vi "gyro app -- V1.vi"() -> ()   [LabVIEW 2020]
uses:
  launch items list.ctl
  pll internal user event action.ctl
  que event bag action.ctl
  server talkto message type.ctl
  server talkback message type.ctl
  cursor action.ctl
panel:
  in  "Main":enum32{"all"}(tab)
  in  "exit!":bool=TRUE
  in  "processes":cluster{"item":T1, "gear":bool}[](array[cluster])=[{"item"=enum."source", "gear"=FALSE}, {"item"=enum."fitter", "gear"=FALSE}, {"item"=enum."sweeper engine", "gear"=FALSE}, {"item"=enum."sweeper monitor", "gear"=FALSE}, {"item"=enum."pll engine", "gear"=FALSE}, {"item"=enum."pll monitor", "gear"=FALSE}]
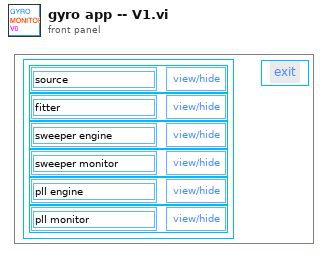
[diagram p1: front panel]
types:
  T1 = typedef "launch items list.ctl" = enum16{"source", "pll engine", "pll monitor", "sweeper engine", "sweeper monitor", "fitter"}
  T2 = typedef "pll internal user event action.ctl" = enum16{"gear pll engine", "start pll async", "stop pll async", "toggle pll async", "gear sweeper", "start sweeper", "stop sweeper", "toggle sweeper", "accept frequency", "reset lorentzian", "accept lorentzian", "update cursors", "pause pll", "unpause pll", "void", "exit", "gear sweeper monitor", "gear sweeper engine", "gear fitter", "gear sourcer", "gear pll monitor"}
  T3 = typedef "que event bag action.ctl" = enum16{"check", "add", "init", "keys", "values"}
  T4 = typedef "server talkback message type.ctl" = cluster{"message":enum16{"new", "void"}}
  T5 = typedef "server talkto message type.ctl" = cluster{"message":enum16{"stop", "start", "update pars", "update request", "new", "launch", "exit", "get", "reset", "pause", "unpause"}}
  T6 = typedef "server talk-to-back pair.ctl" = cluster{"talkback event":refnum<user-event>, "talkto event":refnum<user-event>}
  T7 = typedef "cursor action.ctl" = enum16{"range", "read", "write", "check", "zoom out", "smart zoom out", "zoom to aspect ratio 1", "zoom to win", "zoom out 20%", "zoom in 20%", "-empty", "smart zoom out&aspect", "move range left 20%", "move range right 20%", "move range up 20%", "move range down 20%", "zoom to X win", "zoom to Y win", "zoom out X", "zoom out Y", "zoom in X", "zoom in Y", "check plot scale", "set plot color", "set Xlabel", "set Ylabel", "set cursor color"}
  T8 = enum32{"Invalid", "Standard", "Closed", "Hidden", "Minimized", "Maximized"}
  T9 = typedef "eventvkey.ctl" = enum16{"ASCII", "Enter", "Return", "Shift", "Ctrl", "Alt", "Cmd", "Opt", "Caps", "NumLock", "Clear", "Break", "Up", "Down", "Left", "Right", "Insert", "Delete", "Home", "End", "PageUp", "PageDown", "Escape", "Help", "Pause", "ScrollLock", "F1", "F2", "F3", "F4", "F5", "F6", "F7", "F8", "F9", "F10", "F11", "F12", "F13", "F14", "F15", "F16", "F17", "F18", "F19", "F20", "F21", "F22", "F23", "F24", "Play", "VolumeUp", "VolumeDown", "Mute", "Two Byte Char"}
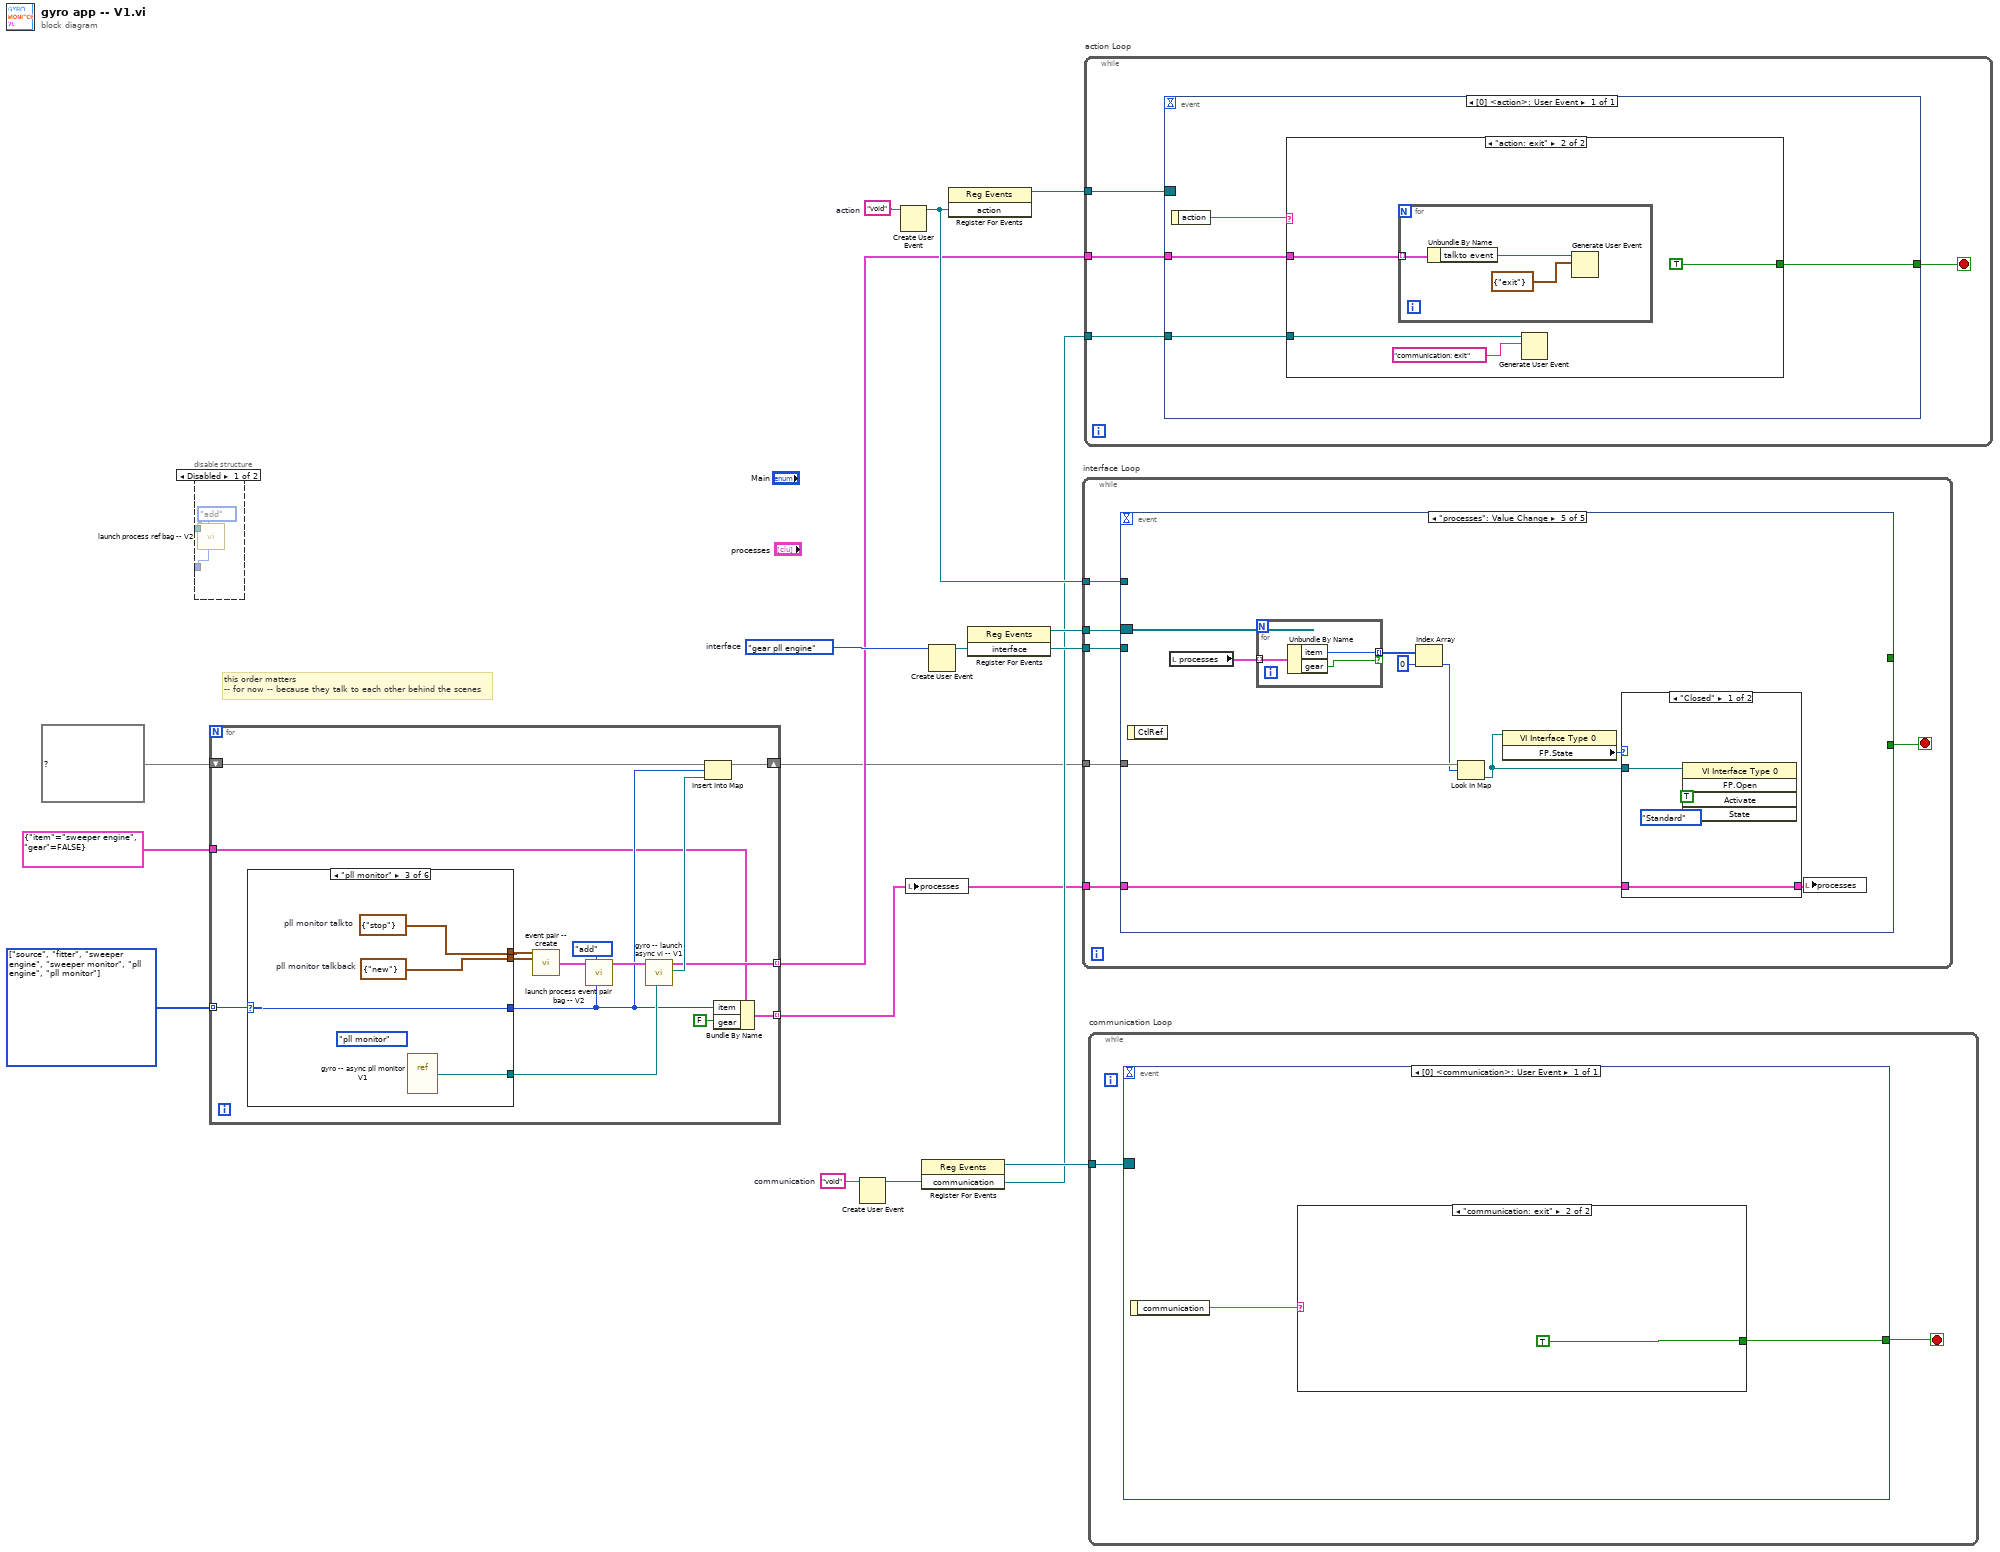
[diagram p0: block diagram]
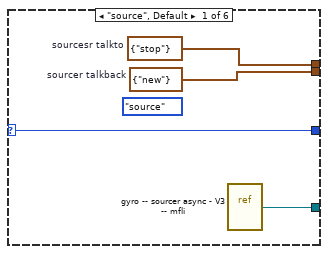
[diagram p3: hidden frame]
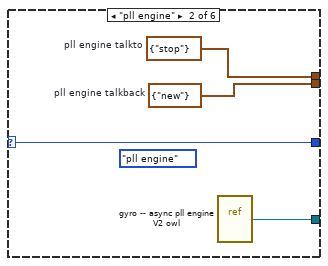
[diagram p4: hidden frame]
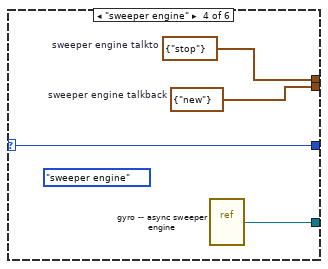
[diagram p5: hidden frame]
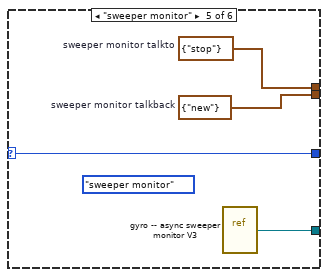
[diagram p6: hidden frame]
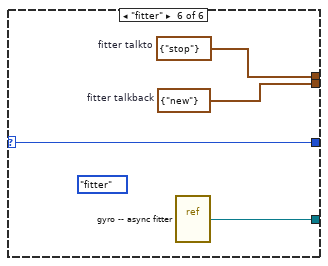
[diagram p7: hidden frame]
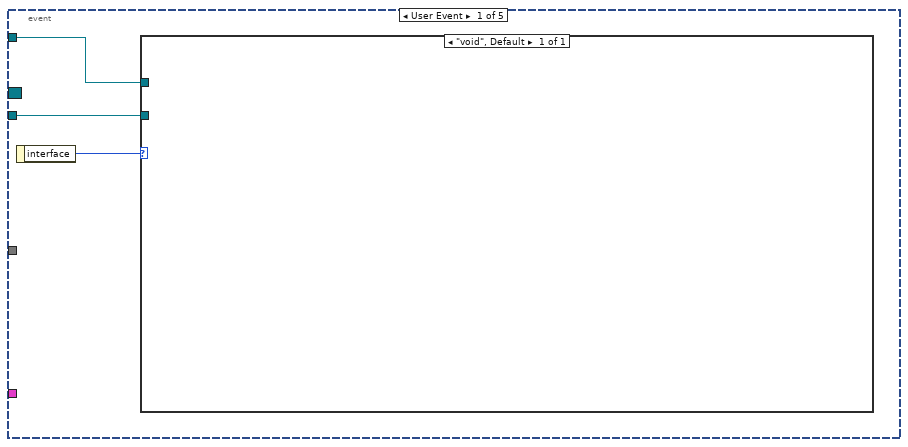
[diagram p10: hidden frame]
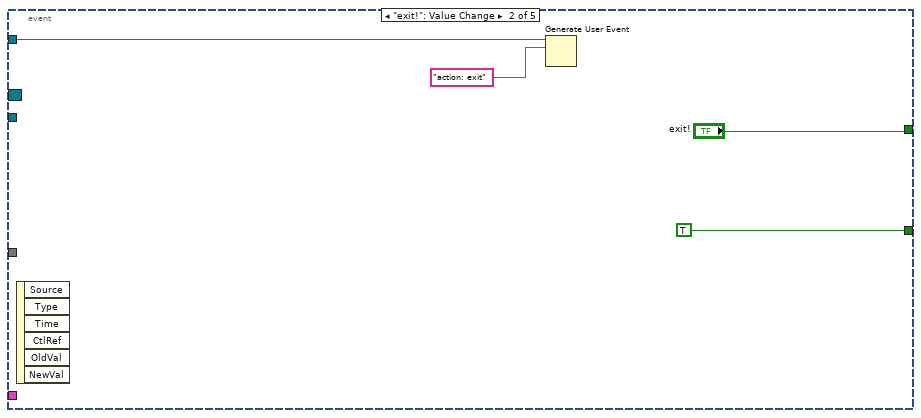
[diagram p11: hidden frame]
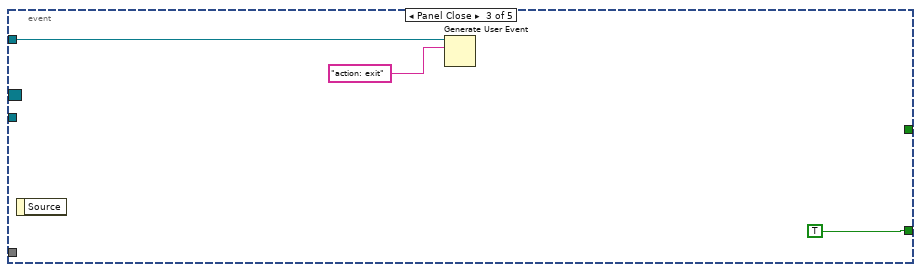
[diagram p12: hidden frame]
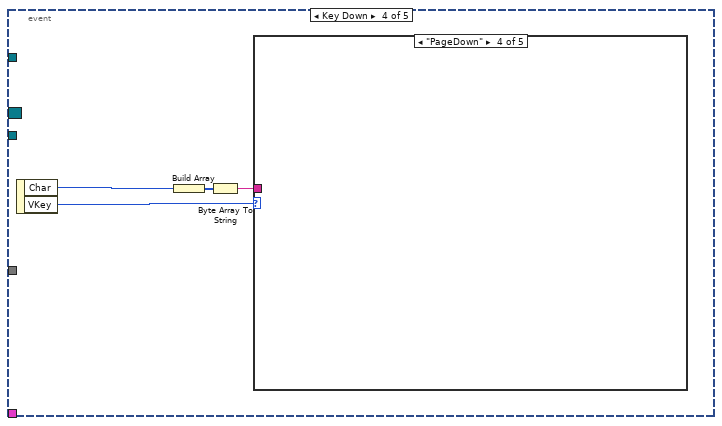
[diagram p13: hidden frame]
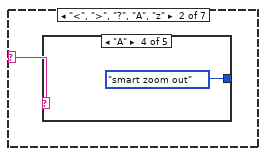
[diagram p16: hidden frame]
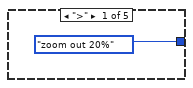
[diagram p17: hidden frame]
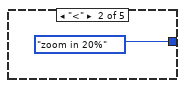
[diagram p18: hidden frame]
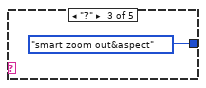
[diagram p19: hidden frame]
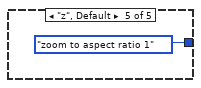
[diagram p20: hidden frame]
diagram:
  w5 = T1[] [enum."source", enum."fitter", enum."sweeper engine", enum."sweeper monitor", enum."pll engine", enum."pll monitor"] items=["source", "pll engine", "pll monitor", "sweeper engine", "sweeper monitor", "fitter"]
  w8 = "void"  # communication
  w11 = "void"  # action
  w13 = pll_internal_user_event_action."gear pll engine"  # interface
  # "this order matters\n-- for now -- because they talk to each other behind the scenes"
  n1 = disable-structure shown="Disabled" {
    disable-tunnel: _ -> [w17 _]
    disable-tunnel: _ -> [w16 _]
    frame Disabled {
      n2 = call "launch process ref bag -- V2.vi"("launch item"=w17, "bag action"=que_event_bag_action."add", "process ref IN"=w16) -> ()  [unwired: 6 in, 3 out]
    }
    frame Enabled {
    }
  }
  n3 = for {
    tunnel: w5 -> [w24] mode=indexing
    tunnel: [w21] -> w7 mode=indexing
    tunnel: [w27] -> w4 mode=indexing
    shift-right: [w25] -> w2
    shift-left: map{T1, refnum<vi>} {} ("Map 2") -> [w26]
    tunnel: cluster{"item":T1, "gear":bool} {"item"=enum."sweeper engine", "gear"=FALSE} ("Cluster") -> [w19]
    n4 = case shown="\"pll monitor\"" w24 {
      selector: w24 -> [w37 w41 w45 w46 w51 w57]
      tunnel: [w35 w39 w43 w49 w53 w56] -> w31
      tunnel: [w34 w38 w42 w48 w52 w55] -> w30
      tunnel: [w37 w41 w45 w46 w51 w57] -> w20
      tunnel: [w36 w40 w44 w47 w50 w54] -> w28
      frame "source", Default {
        (unwired) launch_items_list."source" ("launch items")
        w34 = T4 {"message"=enum."new"}  # sourcer talkback
        w35 = T5 {"message"=enum."stop"}  # sourcesr talkto
        n5 = vi-ref "gyro -- sourcer async - V3 -- mfli.vi"() -> (w36:refnum<vi>)
      }
      frame "pll engine" {
        (unwired) launch_items_list."pll engine" ("launch items")
        w38 = T4 {"message"=enum."new"}  # pll engine talkback
        w39 = T5 {"message"=enum."stop"}  # pll engine talkto
        n6 = vi-ref "gyro -- async pll engine V2 owl.vi"() -> (w40:refnum<vi>)
      }
      frame "pll monitor" {
        (unwired) launch_items_list."pll monitor" ("launch items")
        w42 = T4 {"message"=enum."new"}  # pll monitor talkback
        w43 = T5 {"message"=enum."stop"}  # pll monitor talkto
        n7 = vi-ref "gyro -- async pll monitor V1.vi"() -> (w44:refnum<vi>)
      }
      frame "sweeper engine" {
        (unwired) launch_items_list."sweeper engine" ("launch items")
        w48 = T4 {"message"=enum."new"}  # sweeper engine talkback
        w49 = T5 {"message"=enum."stop"}  # sweeper engine talkto
        n8 = vi-ref "gyro -- async sweeper engine.vi"() -> (w47:refnum<vi>)
      }
      frame "sweeper monitor" {
        (unwired) launch_items_list."sweeper monitor" ("launch items")
        w52 = T4 {"message"=enum."new"}  # sweeper monitor talkback
        w53 = T5 {"message"=enum."stop"}  # sweeper monitor talkto
        n9 = vi-ref "gyro -- async sweeper monitor V3.vi"() -> (w50:refnum<vi>)
      }
      frame "fitter" {
        (unwired) launch_items_list."fitter" ("launch items")
        w55 = T4 {"message"=enum."new"}  # fitter talkback
        w56 = T5 {"message"=enum."stop"}  # fitter talkto
        n10 = vi-ref "gyro -- async fitter.vi"() -> (w54:refnum<vi>)
      }
    }
    n11 = call "event pair -- create.vi"("talkto"=w31, "talkback"=w30) -> ("even pair out"=w29:T6)  [unwired: 11 in, 2 out]
    n12 = call "launch process event pair bag -- V2.vi"("launch item"=w20, "bag action"=que_event_bag_action."add", "event pair IN"=w29) -> ("event pair OUT"=w33:T6)  [unwired: 6 in, 2 out]
    n13 = call "gyro -- launch async vi -- V1.vi"("VI Refnum"=w28, "pll event pair IN"=w33) -> ("reference out"=w22:refnum<vi>, "pll event pair OUT"=w21:T6)  [unwired: 8 in]
    n14 = Insert Into Map(map in=w26, key=w20, value=w22) -> (map out=w25:map{T1, refnum<vi>})  [unwired: 2 out]
    n15 = Bundle By Name(cluster=w19, "item"=w20, "gear"=FALSE) -> (w27:cluster{"item":T1, "gear":bool})
  }
  n16 = Create User Event(user event datatype=w8) -> (user event=w6:refnum<user-event>)  [unwired: 1 in, 1 out]
  n17 = Create User Event(user event datatype=w11) -> (user event=w9:refnum<user-event>)  [unwired: 1 in, 1 out]
  n18 = local write "processes"(w4) -> ()
  n19 = register-events(w6) -> (reference out=w14:refnum<event-registration>)  [unwired: 2 in, 1 out]
  n20 = Create User Event(user event datatype=w13) -> (user event=w12:refnum<user-event>)  [unwired: 1 in, 1 out]
  n21 = register-events(w9) -> (reference out=w10:refnum<event-registration>)  [unwired: 2 in, 1 out]
  n22 = register-events(w12) -> (reference out=w15:refnum<event-registration>)  [unwired: 2 in, 1 out]
  n23 = while "interface Loop" {
    tunnel: w15 -> [w63]
    tunnel: w12 -> [w62]
    tunnel: w9 -> [w60]
    tunnel: w4 -> [w59]
    tunnel: w2 -> [w58]
    stop <- w61 stop-if-true
    n24 = event shown="[4] \"processes\": Value Change" {
      selector: w63 -> [_ _ _ _ _]
      dyn-events: _ -> [_ _ _ _ _]
      timeout: _ -> [_ _ _ _ _]
      tunnel: [_ "exit!" _ _ _] -> _
      tunnel: w62 -> [w65 _ _ _ _]
      tunnel: [_ TRUE TRUE _ _] -> w61
      tunnel: w60 -> [w64 w68 w72 _ _]
      tunnel: w59 -> [_ _ _ _ w93]
      tunnel: w58 -> [_ _ _ _ w92]
      event User Event {
        n25 = event-data() -> ("interface"=w66:T2)  [unwired: 1 in]
        n26 = case shown="\"void\", Default" w66 {
          tunnel: w65 -> [_]
          tunnel: w64 -> [_]
          frame "void", Default {
          }
        }
      }
      event "exit!": Value Change {
        n27 = event-data() -> ()  [unwired: 1 in, 6 out]
        n28 = Generate User Event(user event=w68, event data cluster="action: exit" ("event data")) -> ()  [unwired: 2 in, 2 out]
      }
      event Panel Close {
        n29 = event-data() -> ()  [unwired: 1 in, 1 out]
        n30 = Generate User Event(user event=w72, event data cluster="action: exit" ("event data")) -> ()  [unwired: 2 in, 2 out]
      }
      event Key Down {
        n31 = event-data() -> ("Char"=w75:i16, "VKey"=w77:T9)  [unwired: 1 in]
        n32 = Build Array(w75) -> (w76:i16[])
        n33 = Byte Array To String(unsigned byte array=w76) -> (string=w74:string)
        n34 = case shown="\"PageDown\"" w77 {
          selector: w77 -> [_ _ _ _ w85]
          tunnel: w74 -> [w78 _ _ _ _]
          frame "ASCII", Default {
            n35 = case shown="\"@\"" w78 {
              selector: w78 -> [_ w79 _ _ _ _ _]
              frame "0", Default {
              }
              frame "<", ">", "?", "A", "z" {
                n36 = case shown="\"A\"" w79 {
                  tunnel: [cursor_action."zoom out 20%" ("cursor action") cursor_action."zoom in 20%" ("cursor action") cursor_action."smart zoom out&aspect" ("cursor action") cursor_action."smart zoom out" ("cursor action") cursor_action."zoom to aspect ratio 1" ("cursor action")] -> _
                  frame ">" {
                  }
                  frame "<" {
                  }
                  frame "?" {
                  }
                  frame "A" {
                  }
                  frame "z", Default {
                  }
                }
              }
              frame "r" {
              }
              frame "'", ";", "[", "]", "{", "}" {
              }
              frame "@" {
              }
              frame "#" {
              }
              frame "q" {
              }
            }
          }
          frame "Escape" {
          }
          frame "PageUp" {
          }
          frame "PageDown" {
          }
          frame "Up".."Right" {
            n37 = case shown="\"Down\"" w85 {
              tunnel: [cursor_action."move range right 20%" ("cursor action") cursor_action."move range left 20%" ("cursor action") cursor_action."move range up 20%" ("cursor action") cursor_action."move range down 20%" ("cursor action")] -> _
              frame "Right", Default {
              }
              frame "Left" {
              }
              frame "Up" {
              }
              frame "Down" {
              }
            }
          }
        }
      }
      event "processes": Value Change {
        n38 = event-data() -> ()  [unwired: 1 in, 1 out]
        n39 = local read "processes"() -> (w97:cluster{"item":T1, "gear":bool}[])
        n40 = for {
          tunnel: w97 -> [w101] mode=indexing
          tunnel: [w99] -> w96 mode=indexing if=w100
          n41 = Unbundle By Name(w101) -> ("item"=w99:T1, "gear"=w100:bool)
        }
        n42 = Index Array(array=w96, index=0) -> (element=w90:T1)
        n43 = Look In Map(map=w92, key=w90) -> (value=w91:refnum<vi>)  [unwired: 1 in, 1 out]
        n44 = property class="VI Interface Type 0"(reference=w91) -> ("FP.State"=w98:T8)  [unwired: 1 in, 2 out]
        n45 = case shown="\"Closed\"" w98 {
          tunnel: w91 -> [w105 w107]
          tunnel: [w102 w106] -> w94
          tunnel: w93 -> [w102 w106]
          frame "Closed" {
            n46 = invoke class="VI Interface Type 0" method="FP.Open"(reference=w105, "Activate"=TRUE ("Activate?"), "State"=T8."Standard" ("Front Panel Window:State")) -> ()  [unwired: 2 in, 5 out]
          }
          frame "Standard", Default {
            n47 = invoke class="VI Interface Type 0" method="FP.Close"(reference=w107) -> ()  [unwired: 2 in, 3 out]
          }
        }
        n48 = local write "processes"(w94) -> ()
      }
    }
  }
  n49 = while "action Loop" {
    tunnel: w10 -> [w111]
    tunnel: w7 -> [w109]
    tunnel: w6 -> [w108]
    stop <- w110 stop-if-true
    n50 = event shown="[0] <action>: User Event" {
      selector: w111 -> [_]
      dyn-events: _ -> [_]
      timeout: _ -> [_]
      tunnel: [w114] -> w110
      tunnel: w109 -> [w113]
      tunnel: w108 -> [w112]
      event User Event {
        n51 = event-data() -> ("action"=w115:string)  [unwired: 1 in]
        n52 = case shown="\"action: exit\"" w115 {
          tunnel: [_ TRUE] -> w114
          tunnel: w113 -> [_ w118]
          tunnel: w112 -> [_ w116]
          frame "action: void", Default {
          }
          frame "action: exit" {
            n53 = for {
              tunnel: w118 -> [w120] mode=indexing
              n54 = Unbundle By Name(w120) -> ("talkto event"=w121:refnum<user-event>)
              n55 = Generate User Event(user event=w121, event data cluster=T5 {"message"=enum."exit"} ("event data")) -> ()  [unwired: 2 in, 2 out]
            }
            n56 = Generate User Event(user event=w116, event data cluster="communication: exit" ("event data")) -> ()  [unwired: 2 in, 2 out]
          }
        }
      }
    }
  }
  n57 = while "communication Loop" {
    tunnel: w14 -> [w124]
    stop <- w123 stop-if-true
    n58 = event shown="[0] <communication>: User Event" {
      selector: w124 -> [_]
      dyn-events: _ -> [_]
      timeout: _ -> [_]
      tunnel: [w125] -> w123
      event User Event {
        n59 = event-data() -> ("communication"=w126:string)  [unwired: 1 in]
        n60 = case shown="\"communication: exit\"" w126 {
          tunnel: [_ TRUE] -> w125
          frame "void", Default {
          }
          frame "communication: exit" {
          }
        }
      }
    }
  }
